vi "remove handler (workaround).vi"(8 "error in":errorcluster, 10 "Name":string, 11 "Logger in":refnum<class "Logger.lvclass">) -> (0 "error out":errorcluster, 3 "Logger out":refnum<class "Logger.lvclass">)   [LabVIEW 2024, in "status manager.lvlib"]
uses:
  status manager.lvlib
  <vilib>/Hampel Software Engineering/HSE Logger/Logger/Logger.lvclass
  <vilib>/Hampel Software Engineering/HSE Logger/Handler/Handler.lvclass
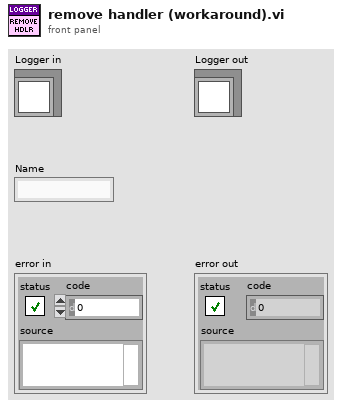
[diagram p1: front panel]
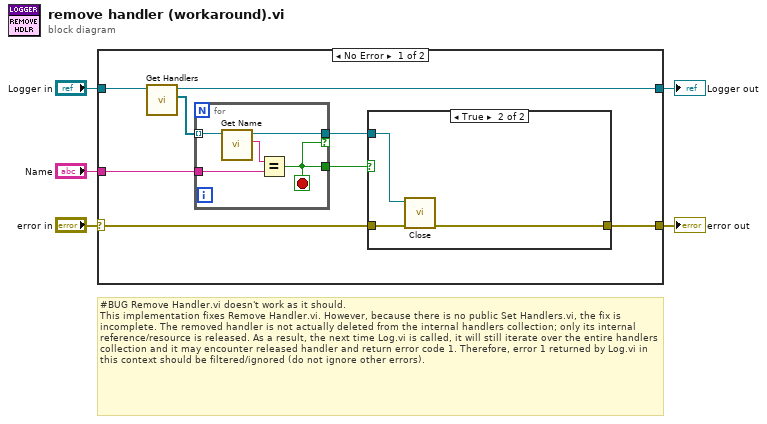
[diagram p0: block diagram]
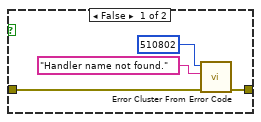
[diagram p2: hidden frame]
diagram:
  # "#BUG Remove Handler.vi doesn't work as it should.\nThis implementation fixes Remove Handler.vi. However, because there is no public Set Handlers.vi, the fix is incomplete. The removed handler is not actually deleted from the internal handlers collection; only its internal reference/resource is released. As a result, the next time Log.vi is called, it will still iterate over the entire handlers collection and it may encounter released handler and return error code 1. Therefore, error 1 returned by Log.vi in this context should be filtered/ignored (do not ignore other errors)."
  n1 = case shown="No Error" "error in" {
    selector: "error in" -> [w13 w27]
    tunnel: [w6 w27] -> w1
    tunnel: [w11 w26] -> w4
    tunnel: "Logger in" -> [w12 w26]
    tunnel: "Name" -> [w9 _]
    frame No Error {
      n2 = call-dynamic "Get Handlers.vi"("Logger in"=w12) -> ("Handlers"=w10:refnum<class "Handler.lvclass">[], "Logger out"=w11:refnum<class "Logger.lvclass">)  [unwired: 8 in, 1 out]
      n3 = for {
        tunnel: w10 -> [w25] mode=indexing
        tunnel: [w24] -> w7 if=w21
        tunnel: w9 -> [w22]
        tunnel: [w21] -> w8
        stop <- w21 stop-if-true
        n4 = call-dynamic "Get Name.vi"("Handler in"=w25) -> ("Name"=w23:string, "Handler out"=w24:refnum<class "Handler.lvclass">)  [unwired: 8 in, 1 out]
        n5 = Equal?(x=w23, y=w22) -> (x = y?=w21:bool)
      }
      n6 = case shown="True" w8 {
        tunnel: w7 -> [_ w20]
        tunnel: w13 -> [w17 w19]
        tunnel: [w16 w18] -> w6
        frame False {
          n7 = call <vilib>:"Error Cluster From Error Code.vi"("error in (no error)"=w17, "error message (\"\")"="Handler name not found.", "error code (0)"=510802) -> ("error out"=w16:errorcluster)  [unwired: 6 in]
        }
        frame True {
          n8 = call-dynamic "Close.vi"("error in"=w19, "Handler in"=w20) -> ("error out"=w18:errorcluster)  [unwired: 8 in, 1 out]
        }
      }
    }
    frame Error {
    }
  }
  "error out" <- w1
  "Logger out" <- w4
